vi "csmdoc_import_VI_description.vi"(8 "error in (no error)":errorcluster, 10 "string":string, 11 "Path":path) -> (0 "error out":errorcluster)   [LabVIEW 2017]
uses:
  Communicable State Machine.lvlib
panel:
  out "Array 2":bool[](array[boolean])
  out "Variant":variant
  out "Array":cluster{"filtered array":string[]}[](array[cluster])
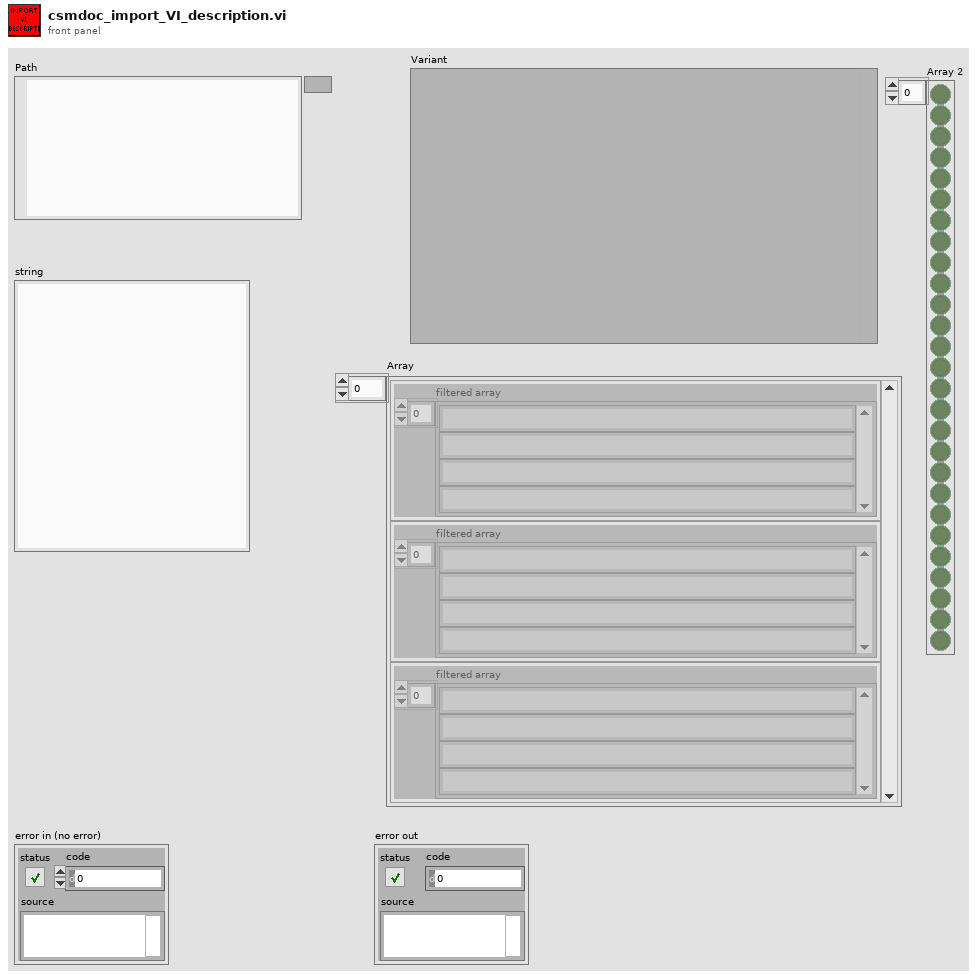
[diagram p1: front panel]
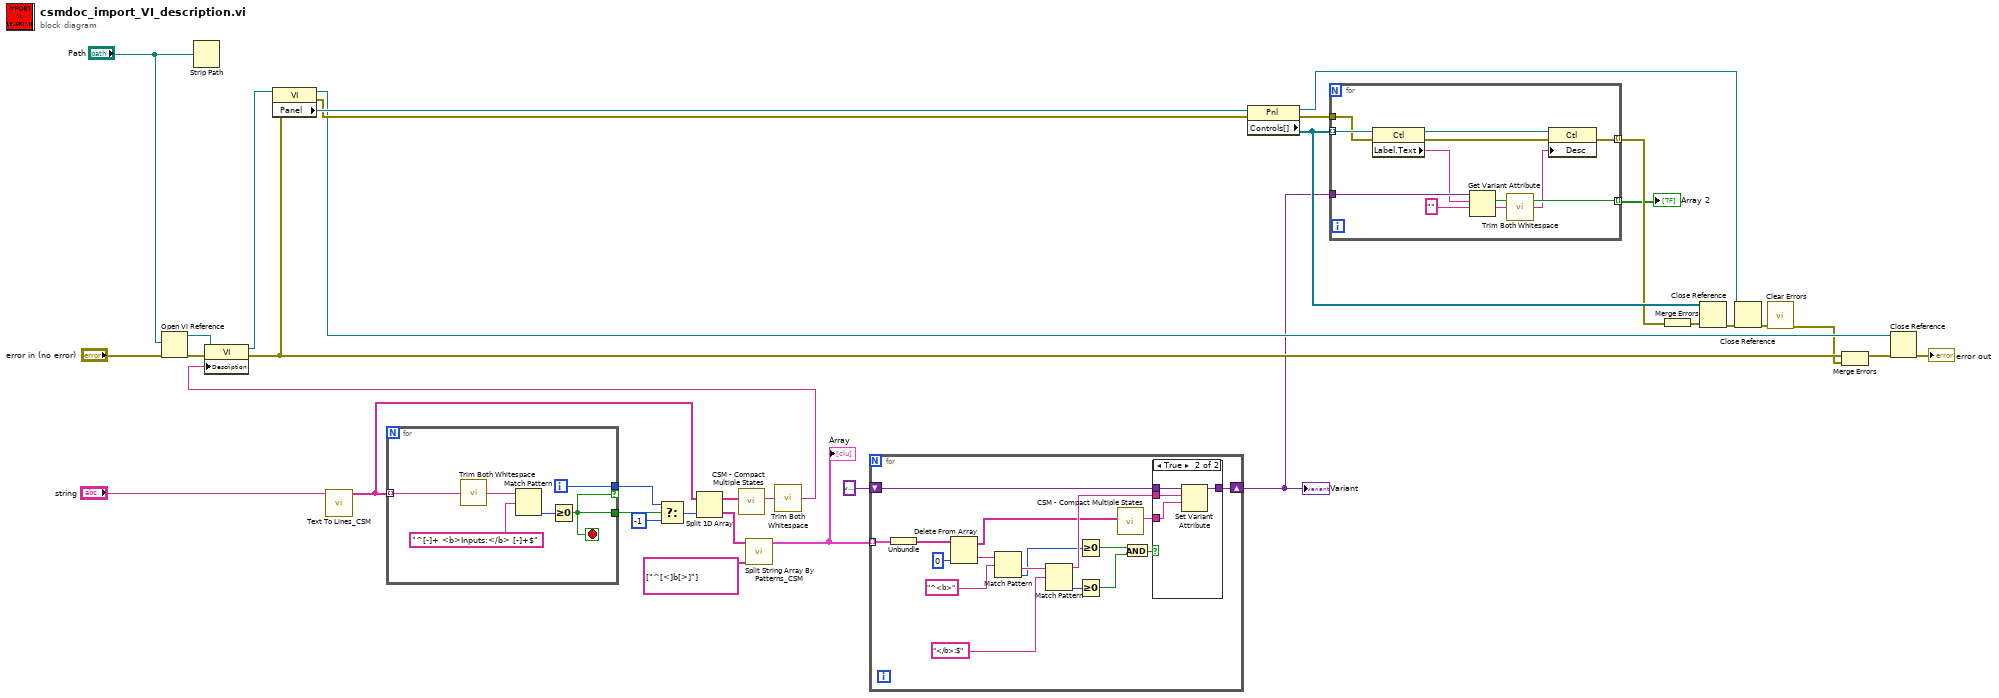
[diagram p0: block diagram]
diagram:
  n1 = Open VI Reference(vi path="Path", error in (no error)="error in (no error)") -> (vi reference=w33:refnum<vi>, error out=w34:errorcluster)  [unwired: 4 in]
  n2 = Strip Path(path="Path") -> ()  [unwired: 2 out]
  n3 = call "Text To Lines_CSM.vi"("string"="string") -> ("Lines"=w12:string[])  [unwired: 9 in, 1 out]
  n4 = for {
    tunnel: w12 -> [w40] mode=indexing
    tunnel: [w36] -> w14 if=w35
    tunnel: [w35] -> w15
    i -> [w36]
    stop <- w35 stop-if-true
    n5 = call "Trim Both Whitespace.vi"("string"=w40) -> ("trimmed string"=w38:string)  [unwired: 1 in]
    n6 = Match Pattern(string=w38, regular expression="^[-]+ <b>Inputs:</b> [-]+$") -> (offset past match=w37:i32)  [unwired: 1 in, 3 out]
    n7 = Greater Or Equal To 0?(x=w37) -> (x >= 0?=w35:bool)
  }
  n8 = Select(t=w14, s=w15, f=-1) -> (s? t:f=w11:i32)
  n9 = Split 1D Array(array=w12, index=w11) -> (first subarray=w3:string[], second subarray=w10:string[])
  n10 = call "CSM - Compact Multiple States.vi"("Multiple States"=w3) -> ("States"=w2:string)  [unwired: 9 in]
  n11 = call "Split String Array By Patterns_CSM.vi"("patterns"=string[] ["^[<]b[>]"], "Text Array"=w10) -> ("Array"=w8:cluster{"filtered array":string[]}[])  [unwired: 9 in]
  "Array" <- w8
  n12 = call "Trim Both Whitespace.vi"("string"=w2) -> ("trimmed string"=w1:string)  [unwired: 1 in]
  n13 = property class="VI"(reference=w33, error in=w34, "Description"=w1) -> (reference out=w32:refnum<vi>, error out=w22:errorcluster)
  n14 = property class="VI"(reference=w32, error in=w22) -> (reference out=w23:refnum<vi>, error out=w30:errorcluster, "Panel"=w31:refnum<vi>)
  n15 = for {
    tunnel: w8 -> [w57] mode=indexing
    shift-right: [w49] -> w6
    shift-left: variant -> [w50]
    n16 = Unbundle(w57) -> ("filtered array"=w56:string[])
    n17 = Delete From Array(array=w56, index=0) -> (deleted portion=w54:string, array with subset deleted=w42:string[])  [unwired: 1 in]
    n18 = Match Pattern(string=w54, regular expression="^<b>" ("delimited string")) -> (after substring=w52:string, offset past match=w46:i32)  [unwired: 1 in, 2 out]
    n19 = Match Pattern(string=w52, regular expression="</b>:$" ("delimited string")) -> (before substring=w48:string, offset past match=w45:i32)  [unwired: 1 in, 2 out]
    n20 = Greater Or Equal To 0?(x=w46) -> (x >= 0?=w44:bool)
    n21 = Greater Or Equal To 0?(x=w45) -> (x >= 0?=w43:bool)
    n22 = call "CSM - Compact Multiple States.vi"("Multiple States"=w42) -> ("States"=w41:string)  [unwired: 9 in]
    n23 = And(x=w44, y=w43) -> (x .and. y?=w47:bool)
    n24 = case shown="True" w47 {
      tunnel: w50 -> [w58 w62]
      tunnel: [w58 w61] -> w49
      tunnel: w48 -> [_ w60]
      tunnel: w41 -> [_ w59]
      frame False {
      }
      frame True {
        n25 = Set Variant Attribute(Variant=w62, name=w60, value=w59) -> (Variant out=w61:variant)  [unwired: 1 in, 2 out]
      }
    }
  }
  "Variant" <- w6
  n26 = property class="Pnl"(reference=w31, error in=w30) -> (reference out=w24:refnum<vi>, error out=w27:errorcluster, "Controls[]"=w29:refnum<vi>[])
  n27 = for {
    tunnel: w29 -> [w73] mode=indexing
    tunnel: w27 -> [w72]
    tunnel: [w69] -> w26 mode=indexing
    tunnel: w6 -> [w68]
    tunnel: [w64] -> w5 mode=indexing
    n28 = property class="Ctl"(reference=w73, error in=w72) -> (reference out=w71:refnum<vi>, error out=w70:errorcluster, "Label.Text"=w67:string)
    n29 = Get Variant Attribute(Variant=w68, name=w67, default value (empty Variant)="" ("regular expression")) -> (found=w64:bool, value=w65:string)  [unwired: 1 in, 2 out]
    n30 = call "Trim Both Whitespace.vi"("string"=w65) -> ("trimmed string"=w63:string)  [unwired: 1 in]
    n31 = property class="Ctl"(reference=w71, error in=w70, "Desc"=w63) -> (error out=w69:errorcluster)  [unwired: 1 out]
  }
  "Array 2" <- w5
  n32 = Merge Errors(w26) -> (w25:errorcluster)
  n33 = Close Reference(reference=w29, error in (no error)=w25) -> (error out=w28:errorcluster)
  n34 = Close Reference(reference=w24, error in (no error)=w28) -> (error out=w21:errorcluster)
  n35 = call <vilib>:"Clear Errors.vi"("error in (no error)"=w21) -> ("error out"=w16:errorcluster)  [unwired: 5 in, 1 out]
  n36 = Merge Errors(w22, w16) -> (w20:errorcluster)
  n37 = Close Reference(reference=w23, error in (no error)=w20) -> (error out=→"error out":errorcluster)
